vi "Conversion_VRMSavg_VRMSdyno.vi"(10 "Dynamic Data":dbl[][](array[numeric]), 11 "VRMS":dbl[][](array[numeric])) -> (0 "VRMS Avg":dbl[](array[numeric]), 3 "VRMS Sine":dbl[][](array[numeric]))   [LabVIEW 2021]
panel:
  out "Column 4":i32
  out "Column 3":i32
  out "Column 2":i32
  out "Column":i32
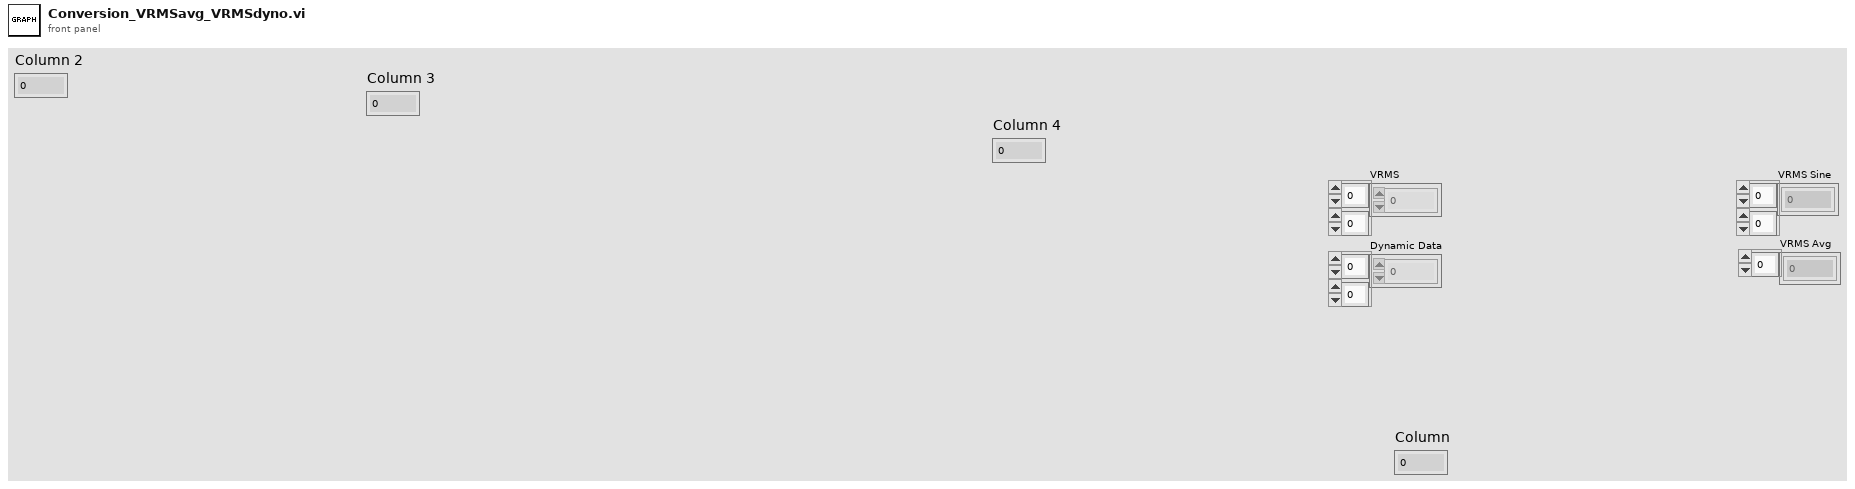
[diagram p1: front panel]
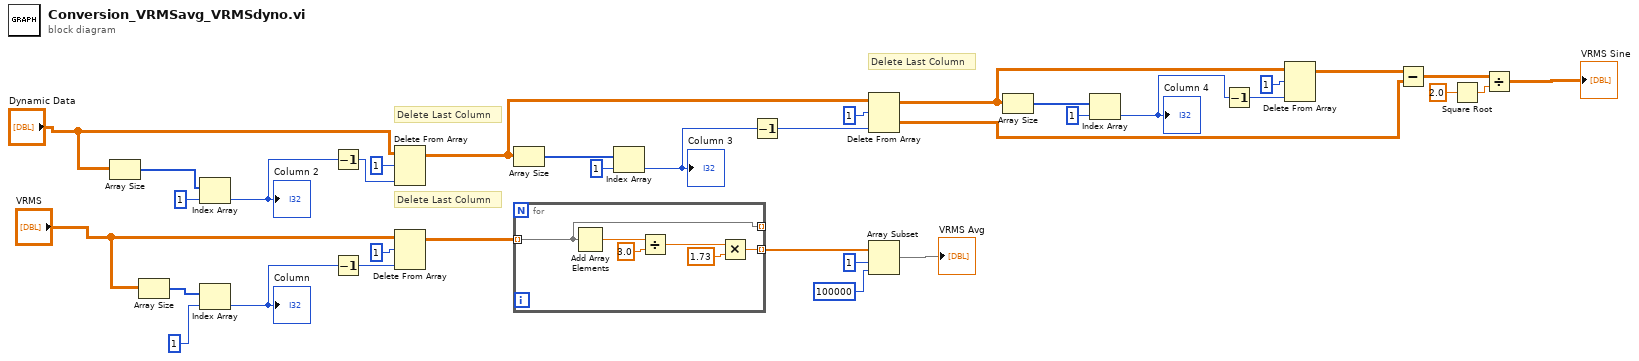
[diagram p0: block diagram]
diagram:
  # "Delete Last Column"
  # "Delete Last Column"
  # "Delete Last Column"
  n1 = Array Size(array="Dynamic Data") -> (size(s)=w26:i32[])
  n2 = Array Size(array="VRMS") -> (size(s)=w35:i32[])
  n3 = Index Array "Index Array"(array=w26, index=1) -> (element=w23:i32)
  "Column 2" <- w23
  n4 = Index Array "Index Array"(array=w35, index=1) -> (element=w32:i32)
  "Column" <- w32
  n5 = Decrement(x=w23) -> (x-1=w22:i32)
  n6 = Decrement(x=w32) -> (x-1=w31:i32)
  n7 = Delete From Array "Delete From Array"(array="Dynamic Data", length=1 ("index (row)"), index (col)=w22) -> (array with subset deleted=w16:dbl[][])  [unwired: 1 in, 1 out]
  n8 = Delete From Array "Delete From Array"(array="VRMS", length=1 ("index (row)"), index (col)=w31) -> (array with subset deleted=w30:dbl[][])  [unwired: 1 in, 1 out]
  n9 = Array Size(array=w16) -> (size(s)=w21:i32[])
  n10 = for {
    tunnel: [w39] -> _ mode=indexing
    tunnel: [w37] -> w27 mode=indexing
    tunnel: w30 -> [w39] mode=indexing
    n11 = Add Array Elements(numeric array=w39) -> (sum=w41:dbl)
    n12 = Divide(x=w41, y=3.0) -> (x/y=w38:dbl)
    n13 = Multiply(x=w38, y=1.73) -> (x*y=w37:dbl)
  }
  n14 = Index Array "Index Array"(array=w21, index=1) -> (element=w18:i32)
  "Column 3" <- w18
  n15 = Decrement(x=w18) -> (x-1=w17:i32)
  n16 = Delete From Array "Delete From Array"(array=w16, length=1 ("index (row)"), index (col)=w17) -> (deleted portion=w6:dbl[][], array with subset deleted=w10:dbl[][])  [unwired: 1 in]
  n17 = Array Subset(array=w27, index=1, length=100000) -> (→"VRMS Avg":dbl[])
  n18 = Array Size(array=w10) -> (size(s)=w15:i32[])
  n19 = Index Array "Index Array"(array=w15, index=1) -> (element=w12:i32)
  "Column 4" <- w12
  n20 = Decrement(x=w12) -> (x-1=w11:i32)
  n21 = Delete From Array "Delete From Array"(array=w10, length=1 ("index (row)"), index (col)=w11) -> (array with subset deleted=w9:dbl[][])  [unwired: 1 in, 1 out]
  n22 = Subtract(x=w9, y=w6) -> (x-y=w8:dbl[][])
  n23 = Square Root(x=2.0) -> (sqrt(x)=w5:dbl)
  n24 = Divide(x=w8, y=w5) -> (x/y=→"VRMS Sine":dbl[][])
